vi "Start.vi"(8 "error in (no error)":errorcluster, 9 "Timeout [ms] (-1)":i32=-1, 11 "Process In":refnum<class "Process.lvclass">) -> (0 "error out":errorcluster, 3 "Process Out":refnum<class "Process.lvclass">)   [LabVIEW 2020, in "Process.lvclass"]
doc: "This VI starts the process which runs asyncronously. The VI blocks the execution until the process has reached its' running state, or the specified timeout expires."
uses:
  Process.lvclass
  Process.lvclass/Process.ctl
  Public/Lifecycle/Lifecycle State.ctl
  <vilib>/Utility/error.llb/Clear Errors.vi
  <vilib>/Utility/error.llb/Error Cluster From Error Code.vi
  <vilib>/ErrorRing/Error Ring.xnode
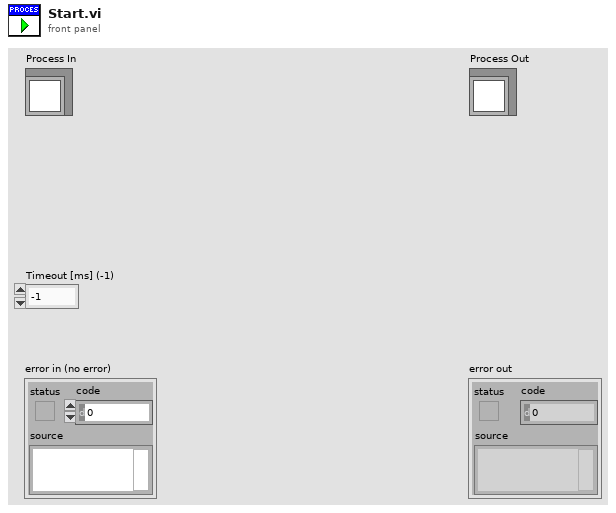
[diagram p1: front panel]
types:
  T1 = typedef "Process.lvclass/Lifecycle State.ctl" = enum16{"Uninitialized", "Initialized", "Started", "Running", "Stopped", "Finished"}
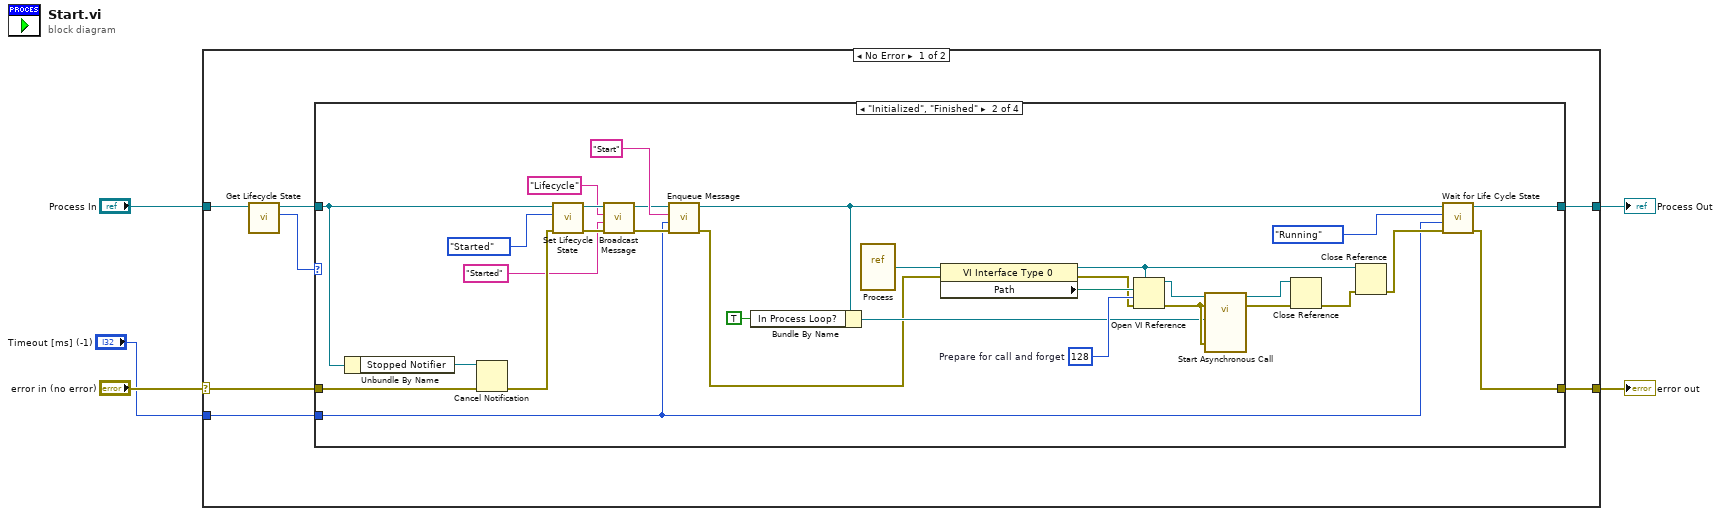
[diagram p0: block diagram]
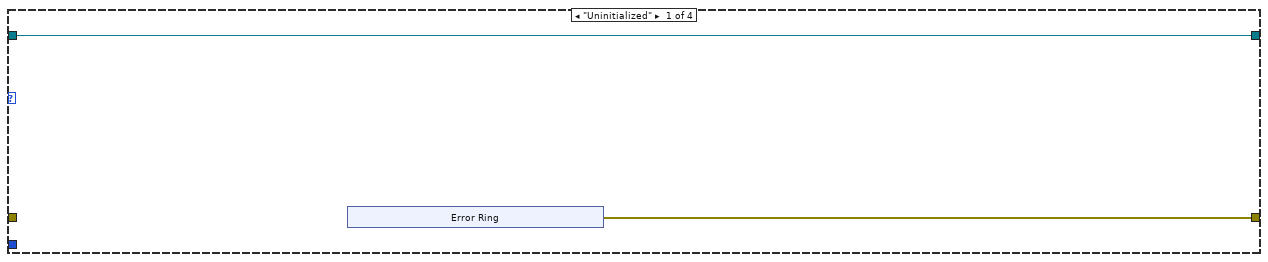
[diagram p2: hidden frame]
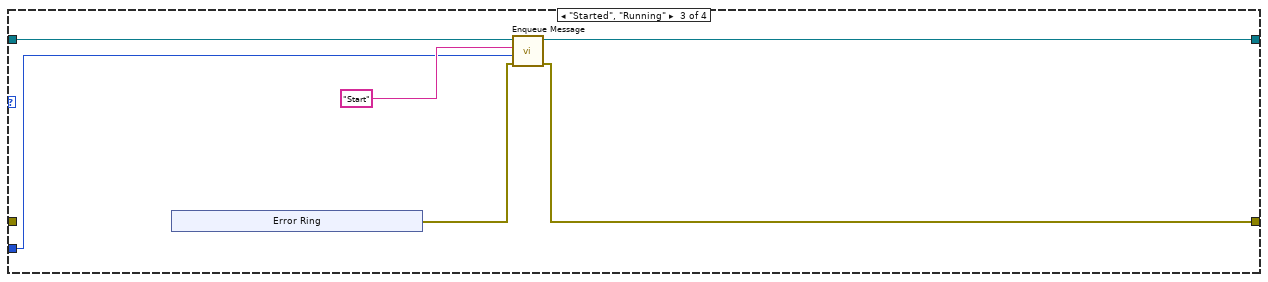
[diagram p3: hidden frame]
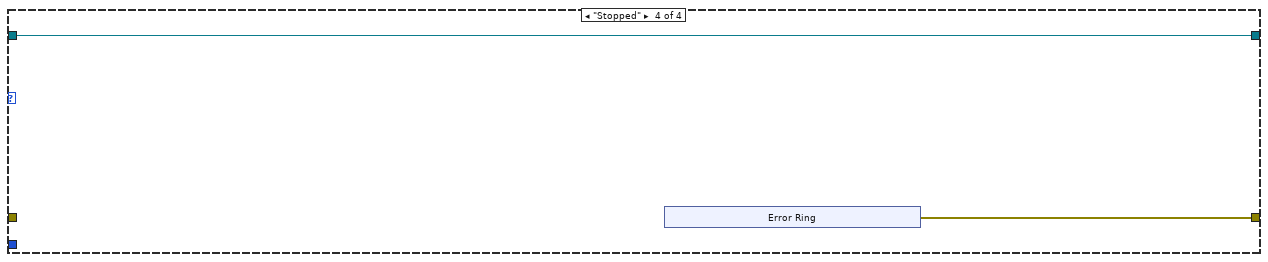
[diagram p4: hidden frame]
diagram:
  n1 = case shown="No Error" "error in (no error)" {
    selector: "error in (no error)" -> [w6 w67]
    tunnel: "Process In" -> [w12 w66]
    tunnel: [w11 w66] -> w4
    tunnel: [w10 w67] -> w3
    tunnel: "Timeout [ms] (-1)" -> [w7 _]
    frame No Error {
      n2 = call "Get Lifecycle State.vi"("Process In"=w12) -> ("Lifecycle State"=w8:T1, "Process Out"=w9:refnum<class "Process.lvclass">)  [unwired: 7 in, 2 out]
      n3 = case shown="\"Initialized\", \"Finished\"" w8 {
        tunnel: [w13 w35 w54 w61] -> w11
        tunnel: [w14 w33 w52 w60] -> w10
        tunnel: w9 -> [w13 w38 w55 w61]
        tunnel: w6 -> [_ w41 _ _]
        tunnel: w7 -> [_ w19 w50 _]
        frame "Uninitialized" {
          n4 = xnode "Error Ring"() -> ("error out"=w14:errorcluster)
        }
        frame "Initialized", "Finished" {
          w46 = 128  # Prepare for call and forget
          n5 = Unbundle By Name(w38) -> ("Stopped Notifier"=w42:refnum<notifier>)
          n6 = Cancel Notification(0:w42, 3:w41) -> (11:w31:errorcluster)  [unwired: 2 out]
          n7 = call "Set Lifecycle State.vi"("error in (no error)"=w31, "Lifecycle State"=Lifecycle_State."Started", "Process In"=w38) -> ("error out"=w26:errorcluster, "Process Out"=w24:refnum<class "Process.lvclass">)  [unwired: 7 in]
          n8 = call-dynamic "Broadcast Message.vi"("error in (no error)"=w26, "Message Data"="Started" ("Message"), "Message"="Lifecycle", "Rig Process In"=w24) -> ("error out"=w25:errorcluster, "Rig Process Out"=w23:refnum<class "Process.lvclass">)  [unwired: 6 in]
          n9 = call "Enqueue Message.vi"("error in (no error)"=w25, "Message Data"=w19, "Message"="Start", "Process In"=w23) -> ("error out"=w37:errorcluster, "Process Out"=w34:refnum<class "Process.lvclass">)  [unwired: 6 in]
          n10 = Bundle By Name(cluster=w34, "In Process Loop?"=TRUE) -> (w39:refnum<class "Process.lvclass">)
          n11 = vi-ref "Process.vi"() -> (w47:refnum<vi>)
          n12 = property class="VI Interface Type 0"(reference=w47, error in=w37) -> (reference out=w29:refnum<vi>, error out=w30:errorcluster, "Path"=w44:path)
          n13 = Open VI Reference(type specifier VI Refnum (for type only)=w29, vi path=w44, options=w46, error in (no error)=w30) -> (vi reference=w45:refnum<vi>, error out=w43:errorcluster)  [unwired: 2 in]
          n14 = call-by-ref "Start Asynchronous Call"(reference=w45, error in=w43, 8:"error in (no error)"=w43, "Process In"=w39) -> (reference out=w49:refnum<vi>, error out=w48:errorcluster)  [unwired: 8 in, 2 out]
          n15 = Close Reference(reference=w49, error in (no error)=w48) -> (error out=w28:errorcluster)
          n16 = Close Reference(reference=w29, error in (no error)=w28) -> (error out=w27:errorcluster)
          n17 = call "Wait for Life Cycle State.vi"("error in (no error)"=w27, "timeout in ms (-1)"=w19, "Lifecycle State"=Lifecycle_State."Running", "Process In"=w34) -> ("error out"=w33:errorcluster, "Process Out"=w35:refnum<class "Process.lvclass">)  [unwired: 5 in, 1 out]
        }
        frame "Started", "Running" {
          n18 = xnode "Error Ring"() -> ("error out"=w53:errorcluster)
          n19 = call "Enqueue Message.vi"("error in (no error)"=w53, "Message Data"=w50, "Message"="Start", "Process In"=w55) -> ("error out"=w52:errorcluster, "Process Out"=w54:refnum<class "Process.lvclass">)  [unwired: 6 in]
        }
        frame "Stopped" {
          n20 = xnode "Error Ring"() -> ("error out"=w60:errorcluster)
        }
      }
    }
    frame Error {
    }
  }
  "error out" <- w3
  "Process Out" <- w4
